vi "RTD_load_preset_dialog.vi"(8 "error in":errorcluster) -> (0 "error out":errorcluster, 1 "failed":bool, 2 "successfull":bool, 3 "preset":T1 {"tref" format="%.3f"; "Rref [Ohm]" format="%.3f"; "RTD poly" format="%_6e"})   [LabVIEW 2020]
uses:
  RTD_preset.ctl
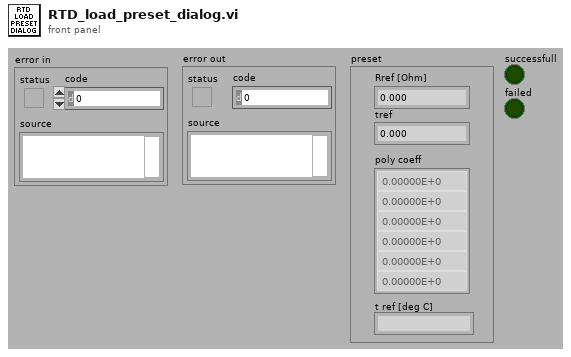
[diagram p1: front panel]
types:
  T1 = typedef "RTD_preset.ctl" = cluster{"Rref [Ohm]":dbl, "tref":dbl, "RTD poly":dbl[], "name":string}
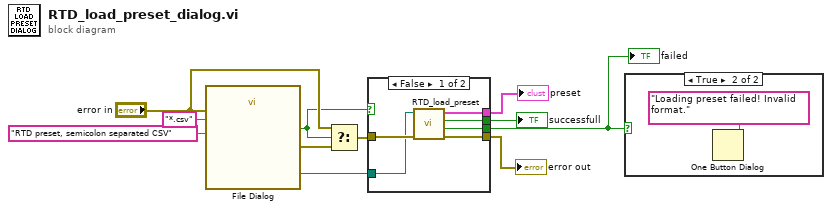
[diagram p0: block diagram]
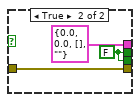
[diagram p3: hidden frame]
diagram:
  n1 = call "File Dialog"("error in"="error in", "pattern (all files)"="*.csv", "pattern label"="RTD preset, semicolon separated CSV") -> ("selected path"=w7:path, "cancelled"=w8:bool, "error out"=w11:errorcluster)  [unwired: 9 in, 1 out]
  n2 = Select(t="error in", s=w8, f=w11) -> (s? t:f=w9:errorcluster)
  n3 = case shown="False" w8 {
    tunnel: w9 -> [w17 w19]
    tunnel: w7 -> [w16 _]
    tunnel: [w15 w19] -> w2
    tunnel: [w14 T1 {"Rref [Ohm]"=0.0, "tref"=0.0, "RTD poly"=[], "name"=""} ("preset")] -> w4
    tunnel: [w13 w20] -> w3
    tunnel: [w12 w20] -> w1
    frame False {
      n4 = call "RTD_load_preset.vi"("error in"=w17, "file path"=w16) -> ("error out"=w15:errorcluster, "failed"=w12:bool, "successfull"=w13:bool, "preset"=w14:T1)  [unwired: 6 in]
    }
    frame True {
      w20 = FALSE ("successfull")
    }
  }
  "preset" <- w4
  "successfull" <- w3
  "failed" <- w1
  "error out" <- w2
  n5 = case shown="True" w1 {
    frame False {
    }
    frame True {
      n6 = One Button Dialog(message="Loading preset failed! Invalid format.") -> ()  [unwired: 1 in, 1 out]
    }
  }
